vi "Przenies dane XY.vi"(7 "Akcja (GET)":T1, 8 "error in (no error)":errorcluster, 9 "Rysuj in":bool, 11 "Wykresy in":string[](array[string])) -> (0 "error out":errorcluster, 1 "Rysuj out":bool, 3 "Wykresy out":string[](array[string]))   [LabVIEW 2014]
doc: "Przenosi aktywnosc rysunku XY"
uses:
  Kontrolki/FVGs/FVG akcje podstawowa.ctl
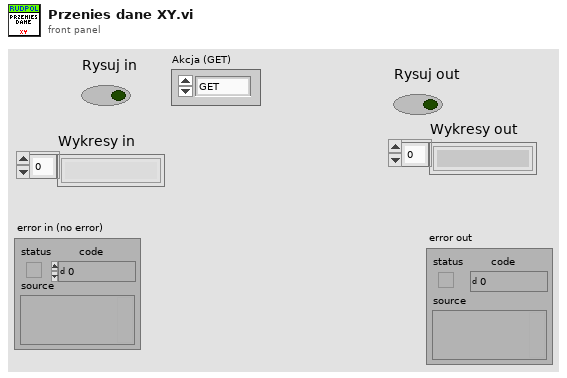
[diagram p1: front panel]
types:
  T1 = typedef "FVG akcje podstawowa.ctl" = enum16{"GET", "SET"}
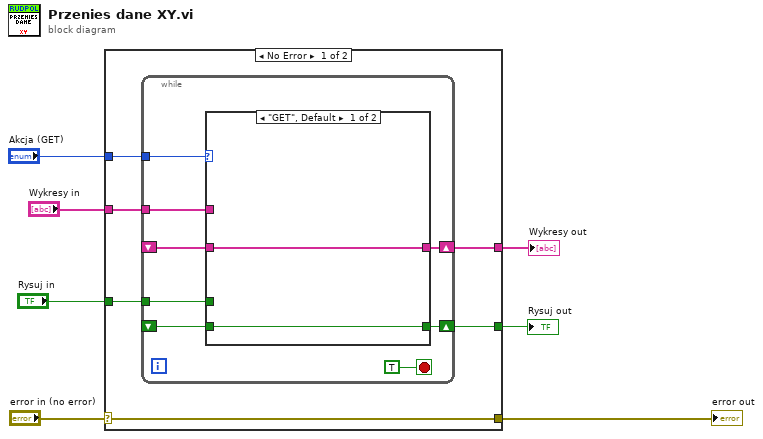
[diagram p0: block diagram]
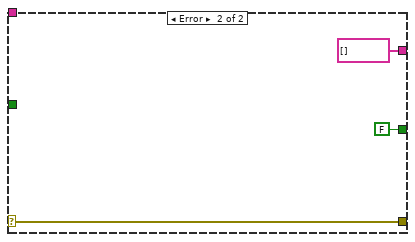
[diagram p3: hidden frame]
diagram:
  n1 = case shown="No Error" "error in (no error)" {
    selector: "error in (no error)" -> [w13 w28]
    tunnel: [w13 w28] -> w6
    tunnel: "Akcja (GET)" -> [w12 _]
    tunnel: "Wykresy in" -> [w11 _]
    tunnel: [w10 string[] [] ("Wykresy in")] -> w3
    tunnel: [w9 FALSE ("Rysuj in")] -> w1
    tunnel: "Rysuj in" -> [w8 _]
    frame No Error {
      n2 = while {
        tunnel: w12 -> [w20]
        tunnel: w11 -> [w18]
        shift-right: [w19] -> w10
        shift-left: _ -> [w15]
        tunnel: w8 -> [w16]
        shift-right: [w17] -> w9
        shift-left: _ -> [w14]
        stop <- TRUE stop-if-true
        n3 = case shown="\"GET\", Default" w20 {
          tunnel: [w23 w25] -> w19
          tunnel: w18 -> [_ w25]
          tunnel: [w22 w24] -> w17
          tunnel: w16 -> [_ w24]
          tunnel: w15 -> [w23 _]
          tunnel: w14 -> [w22 _]
          frame "GET", Default {
          }
          frame "SET" {
          }
        }
      }
    }
    frame Error {
    }
  }
  "error out" <- w6
  "Rysuj out" <- w1
  "Wykresy out" <- w3
